vi "Read Free-throw percentage.vi"(8 "error in (no error)":errorcluster, 11 "Basketball Player in":refnum<class "Basketball Player.lvclass">) -> (0 "error out":errorcluster, 2 "Free-throw percentage":dbl, 3 "Basketball Player out":refnum<class "Basketball Player.lvclass">)   [LabVIEW 2019, in "Basketball Player.lvclass"]
uses:
  Basketball Player.lvclass
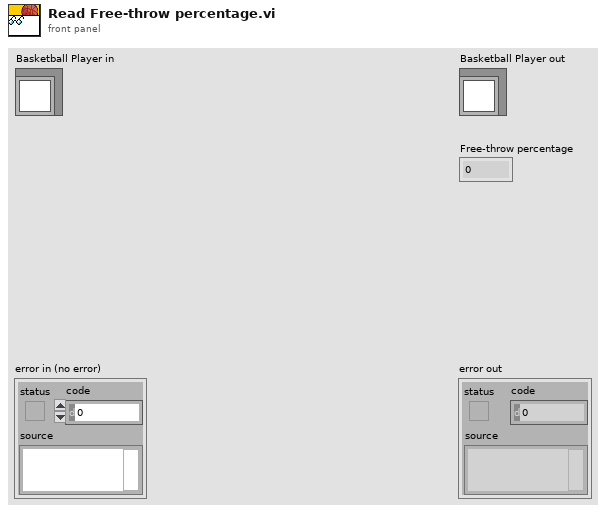
[diagram p1: front panel]
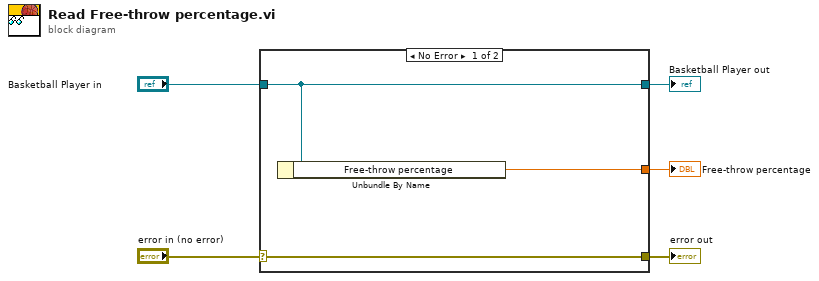
[diagram p0: block diagram]
diagram:
  n1 = case shown="No Error" "error in (no error)" {
    selector: "error in (no error)" -> [w8 w9]
    tunnel: [w8 w9] -> w4
    tunnel: [w7 w10] -> w2
    tunnel: "Basketball Player in" -> [w7 w10]
    tunnel: [w6 _] -> w1
    frame No Error {
      n2 = Unbundle By Name(w7) -> ("Free-throw percentage"=w6:dbl)
    }
    frame Error {
    }
  }
  "error out" <- w4
  "Basketball Player out" <- w2
  "Free-throw percentage" <- w1
